vi "Read AI Terminal Configuration.vi"(8 "error in (no error)":errorcluster, 11 "BNT_ULx-MCSV in":refnum<class "BNT_ULx-MCSV.lvclass">) -> (0 "error out":errorcluster, 2 "AI Terminal Configuration":i32(ring)=-1 items=["default"=-1, "RSE"=10083, "NRSE"=10078, "Differential"=10106, "Pseudodifferential"=12529], 3 "BNT_ULx-MCSV out":refnum<class "BNT_ULx-MCSV.lvclass">)   [LabVIEW 2020, in "BNT_ULx.lvlib" / "BNT_ULx-MCSV.lvclass"]
doc: "Read AI Terminal Configuration."
uses:
  BNT_ULx-MCSV.lvclass
  BNT_ULx-MCSV.lvclass/BNT_ULx-MCSV.ctl
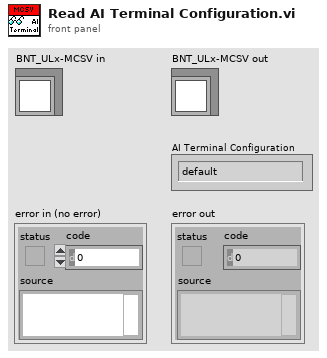
[diagram p1: front panel]
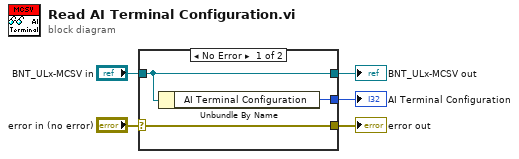
[diagram p0: block diagram]
diagram:
  n1 = case shown="No Error" "error in (no error)" {
    selector: "error in (no error)" -> [w8 w9]
    tunnel: [w8 w9] -> w4
    tunnel: [w7 w10] -> w2
    tunnel: "BNT_ULx-MCSV in" -> [w7 w10]
    tunnel: [w6 _] -> w1
    frame No Error {
      n2 = Unbundle By Name(w7) -> ("AI Terminal Configuration"=w6:i32)
    }
    frame Error {
    }
  }
  "error out" <- w4
  "BNT_ULx-MCSV out" <- w2
  "AI Terminal Configuration" <- w1
